vi "Camera String to Calibration.vi"(8 "error in (no error)":errorcluster, 11 "string in":string) -> (0 "error out":errorcluster, 2 "rectangle":T1 {"Rotation" format="%.2f"; "Left" scale=0.0..1024.0; "Right" scale=0.0..1024.0}, 3 "mm/pixel":dbl)   [LabVIEW 2020]
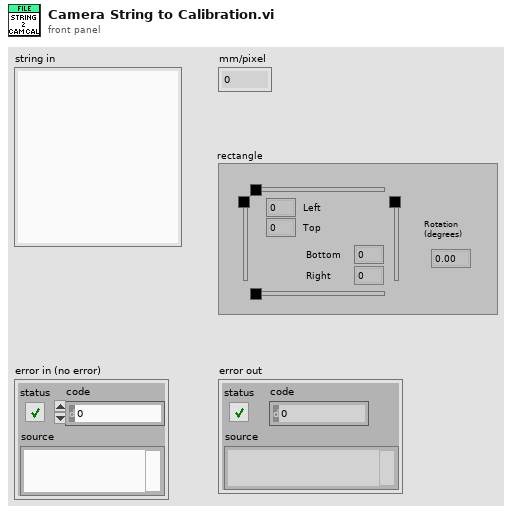
[diagram p1: front panel]
types:
  T1 = typedef "IMAQ Rectangle" = cluster{"Left":i32, "Top":i32, "Right":i32, "Bottom":i32, "Rotation":dbl}
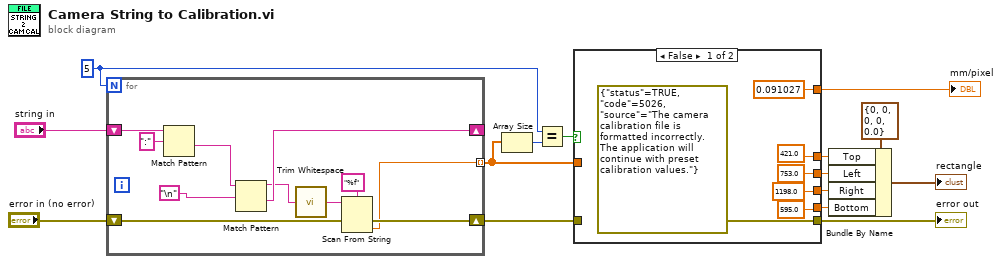
[diagram p0: block diagram]
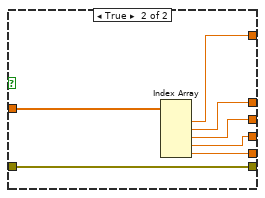
[diagram p2: hidden frame]
diagram:
  w4 = 5
  n1 = for {
    N: w4 -> [_]
    shift-right: [w19] -> _
    shift-left: "string in" -> [w26]
    shift-right: [w22] -> w2
    shift-left: "error in (no error)" -> [w23]
    tunnel: [w21] -> w6 mode=indexing
    n2 = Match Pattern(string=w26, regular expression=":") -> (after substring=w24:string)  [unwired: 1 in, 3 out]
    n3 = Match Pattern(string=w24, regular expression="\n") -> (before substring=w18:string, after substring=w19:string)  [unwired: 1 in, 2 out]
    n4 = call <vilib>:"Trim Whitespace.vi"("string"=w18) -> ("trimmed string"=w17:string)  [unwired: 1 in]
    n5 = Scan From String(format string="%f", input string=w17, error in=w23) -> (error out=w22:errorcluster, output 1=w21:dbl)  [unwired: 2 in, 2 out]
  }
  n6 = Array Size(array=w6) -> (size(s)=w5:i32)
  n7 = Equal?(x=w4, y=w5) -> (x = y?=w1:bool)
  n8 = case shown="False" w1 {
    tunnel: [0.091027 w39] -> w13
    tunnel: [595.0 w38] -> w10
    tunnel: [1198.0 w37] -> w9
    tunnel: [753.0 w36] -> w8
    tunnel: [421.0 w35] -> w7
    tunnel: w6 -> [_ w34]
    tunnel: [errorcluster {"status"=TRUE, "code"=5026, "source"="The camera calibration file is formatted incorrectly. The application will continue with preset calibration values."} ("error in (no error)") w33] -> w3
    tunnel: w2 -> [_ w33]
    frame False {
    }
    frame True {
      n9 = Index Array(array=w34) -> (element #1=w39:dbl, element #2=w35:dbl, element #3=w36:dbl, element #4=w37:dbl, element #5=w38:dbl)  [unwired: 5 in]
    }
  }
  "error out" <- w3
  "mm/pixel" <- w13
  n10 = Bundle By Name(cluster=T1 {"Left"=0, "Top"=0, "Right"=0, "Bottom"=0, "Rotation"=0.0} ("rectangle"), "Top"=w7, "Left"=w8, "Right"=w9, "Bottom"=w10) -> (→"rectangle":T1)
